vi "GPS_StrDismantle_3E2.vi"(1 "LogEvent":refnum<vi>, 2 "VCI_CAN_OBJ_R":T1) -> (0 "GPS位置信息2":T2)   [LabVIEW 2013]
uses:
  Log.ctl
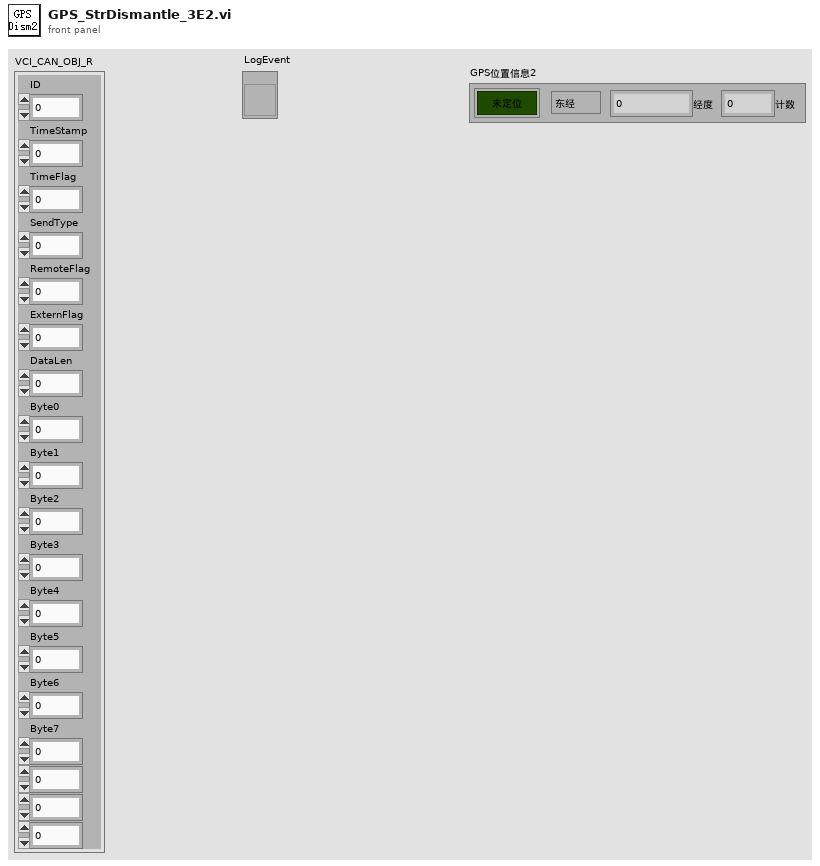
[diagram p1: front panel]
types:
  T1 = cluster{"ID":u32, "TimeStamp":u32, "TimeFlag":u8, "SendType":u8, "RemoteFlag":u8, "ExternFlag":u8, "DataLen":u8, "Byte0":u8, "Byte1":u8, "Byte2":u8, "Byte3":u8, "Byte4":u8, "Byte5":u8, "Byte6":u8, "Byte7":u8, u8, u8, u8}
  T2 = cluster{"经度":u32, "经度状态":enum16{"东经", "西经"}, "定位状态":bool, "计数":u8}
  T3 = typedef "Log.ctl" = cluster{"Event":string, "Value":variant}
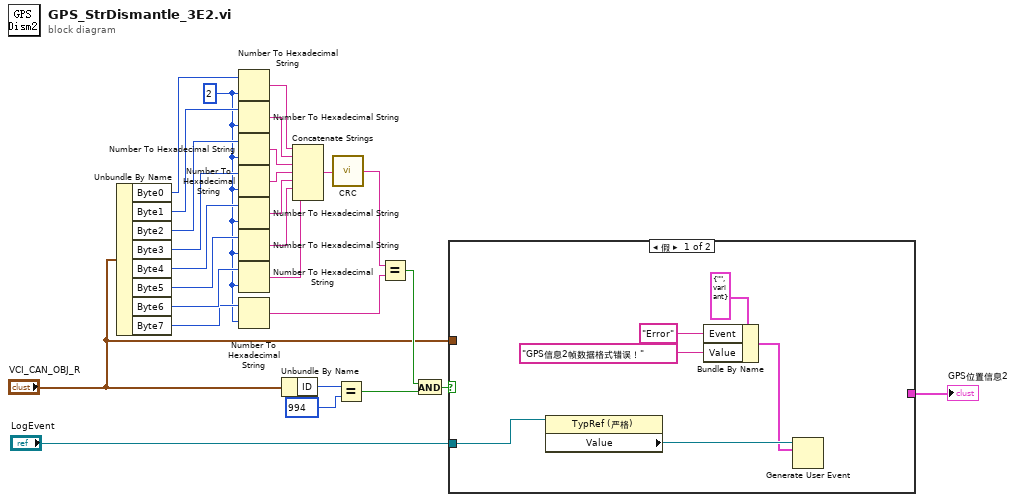
[diagram p0: block diagram]
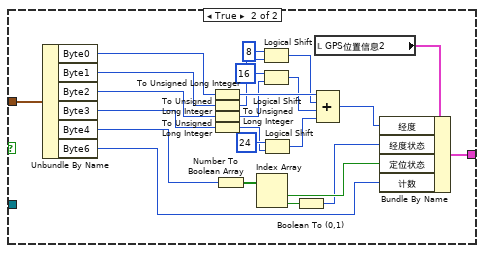
[diagram p2: hidden frame]
diagram:
  w8 = 2
  n1 = Unbundle By Name("VCI_CAN_OBJ_R") -> ("Byte0"=w24:u8, "Byte1"=w23:u8, "Byte2"=w22:u8, "Byte3"=w21:u8, "Byte4"=w20:u8, "Byte5"=w19:u8, "Byte6"=w18:u8, "Byte7"=w9:u8)
  n2 = Number To Hexadecimal String(1:w8, 2:w24) -> (0:w17:string)
  n3 = Number To Hexadecimal String(1:w8, 2:w23) -> (0:w16:string)
  n4 = Number To Hexadecimal String(1:w8, 2:w22) -> (0:w15:string)
  n5 = Number To Hexadecimal String(1:w8, 2:w21) -> (0:w14:string)
  n6 = Number To Hexadecimal String(1:w8, 2:w20) -> (0:w13:string)
  n7 = Number To Hexadecimal String(1:w8, 2:w19) -> (0:w12:string)
  n8 = Number To Hexadecimal String(1:w8, 2:w18) -> (0:w11:string)
  n9 = Number To Hexadecimal String(1:w8, 2:w9) -> (0:w6:string)
  n10 = Unbundle By Name("VCI_CAN_OBJ_R") -> ("ID"=w27:u32)
  n11 = Concatenate Strings(w17, w16, w15, w14, w13, w12, w11) -> (w10:string)
  n12 = call "CRC.vi"("StrIn"=w10) -> ("StrOut"=w7:string)
  n13 = Equal?(x=w27, y=994) -> (x = y?=w3:bool)
  n14 = Equal?(x=w7, y=w6) -> (x = y?=w4:bool)
  n15 = And(x=w4, y=w3) -> (x .and. y?=w5:bool)
  n16 = case shown="假" w5 {
    tunnel: "VCI_CAN_OBJ_R" -> [_ w42]
    tunnel: [_ w34] -> w25
    tunnel: "LogEvent" -> [w28 _]
    frame False {
      n17 = property class="TypRef (严格)"(reference=w28) -> ("Value"=w33:refnum<user-event>)  [unwired: 1 in, 2 out]
      n18 = Bundle By Name(cluster=T3 {"Event"="", "Value"=variant} ("Log"), "Event"="Error", "Value"="GPS信息2帧数据格式错误！" ("消息")) -> (w30:T3)
      n19 = Generate User Event(user event=w33, event data cluster=w30) -> ()  [unwired: 2 in, 2 out]
    }
    frame True {
      n20 = Unbundle By Name(w42) -> ("Byte0"=w41:u8, "Byte1"=w40:u8, "Byte2"=w39:u8, "Byte3"=w38:u8, "Byte4"=w37:u8, "Byte6"=w35:u8)
      n21 = To Unsigned Long Integer(number=w41) -> (unsigned 32bit integer=w57:u32)
      n22 = To Unsigned Long Integer(number=w40) -> (unsigned 32bit integer=w56:u32)
      n23 = To Unsigned Long Integer(number=w39) -> (unsigned 32bit integer=w53:u32)
      n24 = To Unsigned Long Integer(number=w38) -> (unsigned 32bit integer=w51:u32)
      n25 = Number To Boolean Array(number=w37) -> (Boolean array=w46:bool[])
      n26 = Index Array(array=w46) -> (element #1=w45:bool, element #2=w44:bool)  [unwired: 2 in]
      n27 = Logical Shift(y=u8 8, x=w56) -> (x << y=w50:u32)
      n28 = Logical Shift(y=u8 16, x=w53) -> (x << y=w49:u32)
      n29 = Logical Shift(y=u8 24, x=w51) -> (x << y=w48:u32)
      n30 = Boolean To (0,1)(Boolean=w44) -> (0, 1=w43:i16)
      n31 = local read "GPS位置信息2"() -> (w36:T2)
      n32 = Compound Arithmetic op=ADD(w57, w50, w49, w48) -> (w47:u32)
      n33 = Bundle By Name(cluster=w36, "经度"=w47, "经度状态"=w43, "定位状态"=w45, "计数"=w35) -> (w34:T2)
    }
  }
  "GPS位置信息2" <- w25
